vi "Address Message.vi"(8 "Message Priority (Normal)":T1=enum."Normal", 9 "Message":refnum<class "Message.lvclass">, 10 "Destination":refnum<class "Message Enqueuer.lvclass">) -> (3 "Self-Addressed Message":refnum<class "Self-Addressed Msg.lvclass">)   [LabVIEW 2020, in "Self-Addressed Msg.lvclass"]
doc: "This message is <b>DEPRECATED</b>. Please replace it with <b>Actor Framework.lvlib:Self-Addressed Msg.lvclass</b>, which provides the same functionality and a cleaner PPL build experience.\n\n<p>(<strong>Filename</strong>: <span class=\"dnl\">Actor Framework.lvlib:Self-Addressed Msg.lvclass:Address Message.vi</span>)</p>\n\n<p>Creates a self-addressed message by storing an enqueuer inside a message. Later, when you send the message with the <a href=\"nihelplauncher://docs/csh?context=lvcore_lvcomm_af_send_sam\">Send Self-Addressed Message</a> method, the message will be sent to the actor that uses this enqueuer.</p>"
uses:
  Self-Addressed Msg.lvclass
  Message/Message.lvclass
  Message Enqueuer/Message Enqueuer.lvclass
  Self-Addressed Msg.lvclass/Self-Addressed Msg.ctl
  Message Enqueuer/Message Priority.ctl
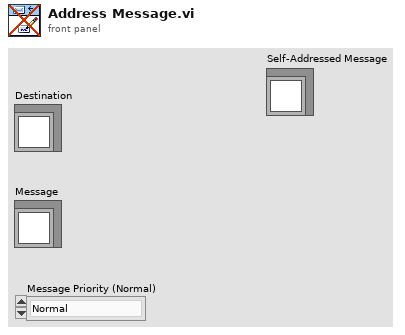
[diagram p1: front panel]
types:
  T1 = typedef "Actor Framework.lvlib/Message Enqueuer.lvclass/Message Priority.ctl" = enum16{"Low", "Normal", "High"}
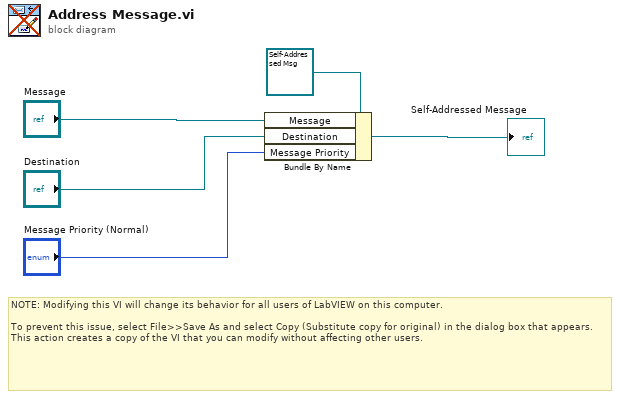
[diagram p0: block diagram]
diagram:
  # "NOTE: Modifying this VI will change its behavior for all users of LabVIEW on this computer.\n\nTo prevent this issue, select File>>Save As and select Copy (Substitute copy for original) in the dialog box that appears. This action creates a copy of the VI that you can modify without affecting other users."
  n1 = Bundle By Name(cluster=refnum<class "Self-Addressed Msg.lvclass"> refnum ("Self-Addressed Message in"), "Message"="Message", "Destination"="Destination", "Message Priority"="Message Priority (Normal)") -> (→"Self-Addressed Message":refnum<class "Self-Addressed Msg.lvclass">)
